vi "Acquire and enque.vi"(8 "error in (no error)":errorcluster, 10 "Data In":T1, 11 "Queue in":refnum<queue>) -> (0 "error out":errorcluster, 2 "Data Out":T1)   [LabVIEW 2015]
uses:
  TypeDefs/Acq Loop Data.ctl
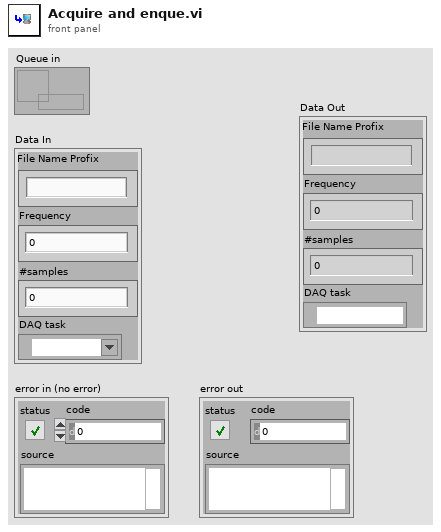
[diagram p1: front panel]
types:
  T1 = typedef "Acq Loop Data.ctl" = cluster{"File Name Profix":string, "Frequency":dbl, "#samples":i32, "DAQ task ":refnum<k21>}
  T2 = typedef "Queue Data" = cluster{"Action":string, "Data":dbl[]}
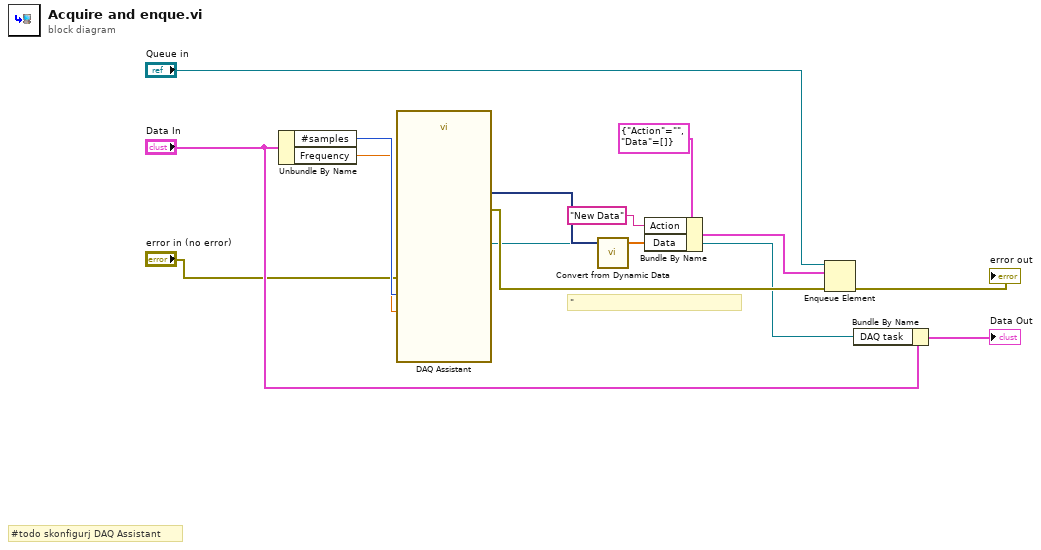
[diagram p0: block diagram]
diagram:
  # "#todo skonfigurj DAQ Assistant"
  # "\""
  n1 = Unbundle By Name("Data In") -> ("#samples"=w7:i32, "Frequency"=w6:dbl)
  n2 = call "DAQ Assistant"("rate"=w6, "number of samples"=w7, "error in"="error in (no error)") -> ("task out"=w1:refnum<k21>, "data"=w3:dynamicdata, "error out"=w4:errorcluster)  [unwired: 13 in, 1 out]
  n3 = call "Convert from Dynamic Data"("Dynamic Data Type"=w3) -> ("Array"=w2:dbl[])  [unwired: 3 in]
  n4 = Bundle By Name(cluster=T2 {"Action"="", "Data"=[]}, "Action"="New Data", "Data"=w2) -> (w10:T2)
  n5 = Enqueue Element(queue="Queue in", element=w10, error in (no error)=w4) -> (error out=→"error out":errorcluster)  [unwired: 1 in, 2 out]
  n6 = Bundle By Name(cluster="Data In", "DAQ task"=w1) -> (→"Data Out":T1)
